vi "Shooter Camera Distance.vi"() -> (1 "Target Found?":bool, 2 "Yaw":dbl, 3 "Distance (ft)":dbl)   [LabVIEW 2016]
uses:
  <vilib>/Rock Robotics/Network Tables/NT Read Number.vi
panel:
  in  "Debug Yaw":dbl
  in  "Debug Distance":dbl
  in  "Debug Target Found":bool
  in  "Debug?":bool
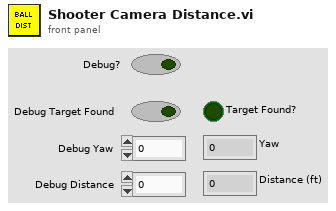
[diagram p1: front panel]
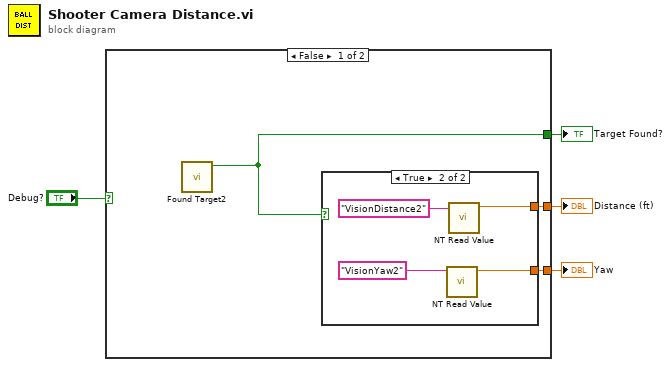
[diagram p0: block diagram]
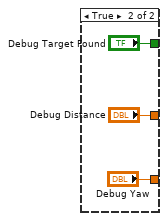
[diagram p3: hidden frame]
diagram:
  n1 = case shown="False" "Debug?" {
    tunnel: [w7 "Debug Distance"] -> w4
    tunnel: [w5 "Debug Target Found"] -> w3
    tunnel: [w6 "Debug Yaw"] -> w2
    frame False {
      n2 = call "Found Target2.vi"() -> ("Boolean"=w5:bool)  [unwired: 11 in]
      n3 = case shown="True" w5 {
        tunnel: [_ w10] -> w7
        tunnel: [_ w8] -> w6
        frame False {
        }
        frame True {
          n4 = call-poly <vilib>:"NT Read Value.vi"("Name"="VisionYaw2") -> ("Numeric"=w8:dbl)  [unwired: 9 in, 1 out]
          n5 = call-poly <vilib>:"NT Read Value.vi"("Name"="VisionDistance2") -> ("Numeric"=w10:dbl)  [unwired: 9 in, 1 out]
        }
      }
    }
    frame True {
    }
  }
  "Distance (ft)" <- w4
  "Target Found?" <- w3
  "Yaw" <- w2
